vi "Generate Training Sample (RNN).vi"(2 "iteration":i32, 3 "seg_length":i32, 4 "indices":i64[](array[numeric])) -> (0 "targets":i64[](array[numeric]), 1 "inputs":i64[](array[numeric]))   [LabVIEW 2014]
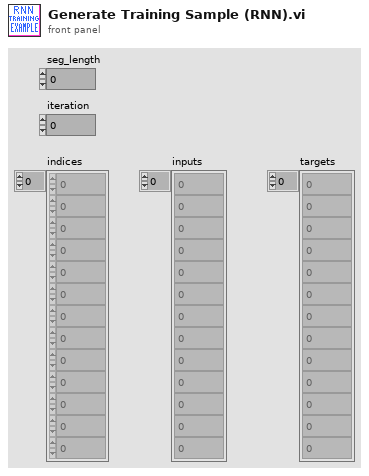
[diagram p1: front panel]
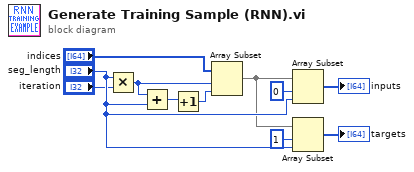
[diagram p0: block diagram]
diagram:
  n1 = Multiply(x="seg_length", y="iteration") -> (x*y=w2:i32)
  n2 = Add(x=w2, y="seg_length") -> (x+y=w3:i32)
  n3 = Increment(x=w3) -> (x+1=w4:i32)
  n4 = Array Subset(array="indices", index=w2, length=w4) -> (w5:i64[])
  n5 = Array Subset(array=w5, index=0, length="seg_length") -> (→"inputs":i64[])
  n6 = Array Subset(array=w5, index=1, length="seg_length") -> (→"targets":i64[])
